vi "SLSC Get IP Address from Chassis.vi"(8 "error in (no error)":errorcluster, 10 "IP Address Global Name":string, 11 "Parent Ref":T1 format="%.0x") -> (0 "error out":errorcluster, 1 "Chassis ID Type":i32(ring) items=["ChassisName", "HostnameIPAddress"], 2 "Name or IP Address":string, 3 "Item Ref out":T1 format="%.0x")   [LabVIEW 2015, in "SLSC CD System Explorer.lvlib"]
uses:
  SLSC CD System Explorer.lvlib
  <vilib>/NI Veristand/Custom Device API/Custom Device Item Ref.ctl
  <vilib>/NI Veristand/Custom Device API/Get Item Property (String).vi
  <vilib>/NI VeriStand/Custom Device API/Custom Device API.lvlib
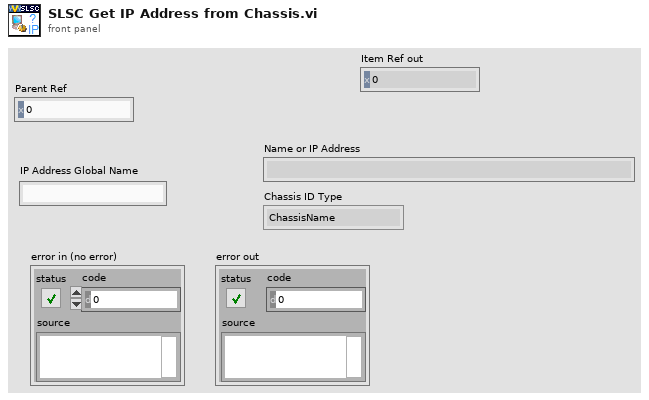
[diagram p1: front panel]
types:
  T1 = typedef "Custom Device API.lvlib/Custom Device Item Ref.ctl" = u64
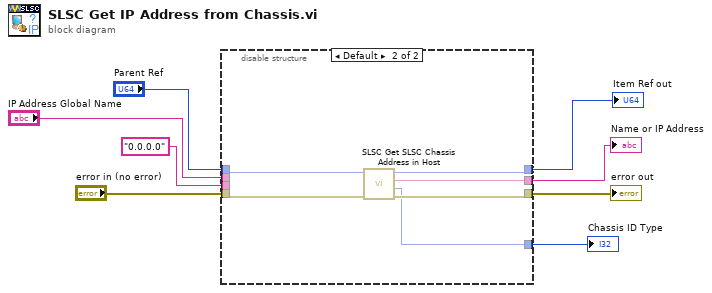
[diagram p0: block diagram]
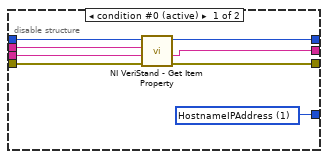
[diagram p2: hidden frame]
diagram:
  n1 = disable-structure shown="Default" {
    disable-tunnel: [w16 w19] -> w8
    disable-tunnel: [w15 w18] -> w7
    disable-tunnel: "0.0.0.0" ("Default Value") -> [w14 _]
    disable-tunnel: "Parent Ref" -> [w13 w22]
    disable-tunnel: "error in (no error)" -> [w12 w21]
    disable-tunnel: [w11 w20] -> w3
    disable-tunnel: "IP Address Global Name" -> [w10 _]
    disable-tunnel: [w9 w17] -> w1
    frame condition #0 (active) {
      w9 = 1 items=["ChassisName", "HostnameIPAddress"] ("ChassisIDType")
      n2 = call-poly <vilib>:"NI VeriStand - Get Item Property.vi"("error in (no error)"=w12, "Default Value"=w14, "Property Name"=w10, "Item Ref in"=w13) -> ("error out"=w15:errorcluster, "Value"=w16:string, "Item Ref out"=w11:T1)  [unwired: 4 in, 1 out]
    }
    frame condition #1 {
      n3 = call "SLSC Get SLSC Chassis Address in Host.vi"("error in (no error)"=w21, "Parent Ref"=w22) -> ("error out"=w18:errorcluster, "ChassisIDType"=w17:i32, "IP Address"=w19:string, "Item Ref out"=w20:T1)  [unwired: 6 in]
    }
  }
  "Name or IP Address" <- w8
  "error out" <- w7
  "Item Ref out" <- w3
  "Chassis ID Type" <- w1
